vi "Mean and Standard Deviation.vi"() -> ()   [LabVIEW 2012]
panel:
  in  "Knob":dbl(knob) scale=10.0..500.0
  out "While Loop Counter":dbl
  in  "Stop Button":bool
  out "Waveform Chart":cluster{"number: 0 to 1":dbl, dbl, dbl}(graph)
  # "Frequency In Milliseconds"
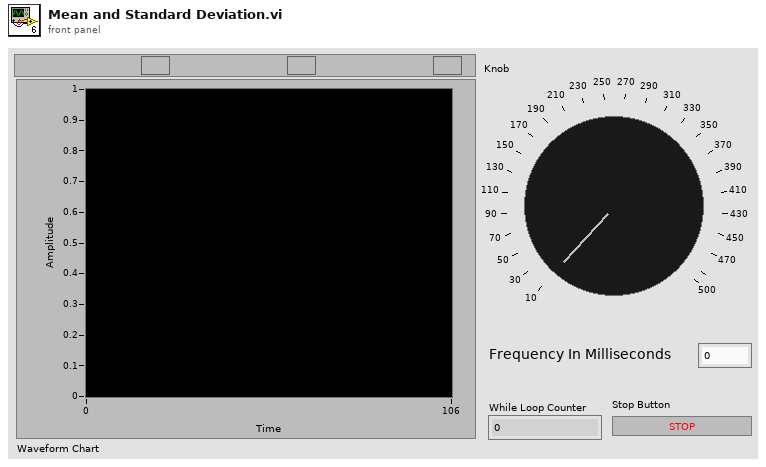
[diagram p1: front panel]
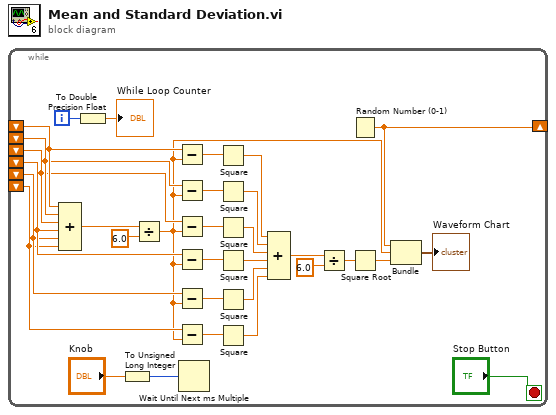
[diagram p0: block diagram]
diagram:
  n1 = while {
    shift-right: [w25] -> _
    shift-left: _ -> [w23]
    shift-left: _ -> [w2]
    shift-left: _ -> [w3]
    shift-left: _ -> [w4]
    shift-left: _ -> [w6]
    shift-left: _ -> [w5]
    i -> [w29]
    stop <- "Stop Button" stop-if-true
    n2 = Compound Arithmetic op=ADD(w23, w6, w5, w4, w3, w2) -> (w27:dbl)
    n3 = To Double Precision Float(number=w29) -> (double precision float=→"While Loop Counter":dbl)
    n4 = To Unsigned Long Integer(number="Knob") -> (unsigned 32bit integer=w30:u32)
    n5 = Divide(x=w27, y=6.0) -> (x/y=w1:dbl)
    n6 = Subtract(x=w23, y=w1) -> (x-y=w22:dbl)
    n7 = Subtract(x=w6, y=w1) -> (x-y=w11:dbl)
    n8 = Subtract(x=w5, y=w1) -> (x-y=w10:dbl)
    n9 = Subtract(x=w4, y=w1) -> (x-y=w9:dbl)
    n10 = Subtract(x=w3, y=w1) -> (x-y=w8:dbl)
    n11 = Subtract(x=w2, y=w1) -> (x-y=w7:dbl)
    n12 = Wait Until Next ms Multiple(millisecond multiple=w30) -> ()  [unwired: 1 out]
    n13 = Square(x=w22) -> (x^2=w21:dbl)
    n14 = Square(x=w11) -> (x^2=w20:dbl)
    n15 = Square(x=w10) -> (x^2=w19:dbl)
    n16 = Square(x=w9) -> (x^2=w18:dbl)
    n17 = Square(x=w8) -> (x^2=w17:dbl)
    n18 = Square(x=w7) -> (x^2=w16:dbl)
    n19 = Compound Arithmetic op=ADD(w21, w20, w19, w18, w17, w16) -> (w15:dbl)
    n20 = Divide(x=w15, y=6.0) -> (x/y=w13:dbl)
    n21 = Random Number (0-1)() -> (number: 0 to 1=w25:dbl)
    n22 = Square Root(x=w13) -> (sqrt(x)=w12:dbl)
    n23 = Bundle("number: 0 to 1"=w25, w1, w12) -> (→"Waveform Chart":cluster{"number: 0 to 1":dbl, dbl, dbl})  [unwired: 1 in]
  }
